vi "Loop.vi"(9 "Error Queue":refnum<queue>, 10 "Event Actor Queue":refnum<queue>, 11 "Dev Actor Panel":refnum<class "Dev Panel.lvclass">) -> ()   [LabVIEW 2021, in "Dev Panel.lvclass"]
uses:
  Dev Panel.lvclass
  C:/git/jettl/src/Event Actor/Event Actor.lvclass
  Actor/Event Actor/Event Actor.lvclass
  Dev Panel.lvclass/Dev Panel.ctl
  Actor/Msgs/Teardown/Teardown Msg/Teardown Msg.lvclass
  C:/git/jettl/src/Actor/Msg/Msg.lvclass
  Msgs/Pop Up/Pop Up Msg/Pop Up Msg.lvclass
  Actor/Msgs/Merge Error/Merge Error Msg/Merge Error Msg.lvclass
panel:
  in  "Button":bool
  out "String Indicator":string
  in  "Pop Up":bool
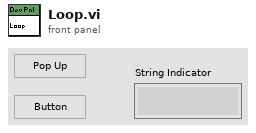
[diagram p1: front panel]
types:
  T1 = cluster{"Teardown":refnum<user-event>, "Pop Up":refnum<user-event>, "String Indicator":refnum<user-event>, "Button":refnum<user-event>}
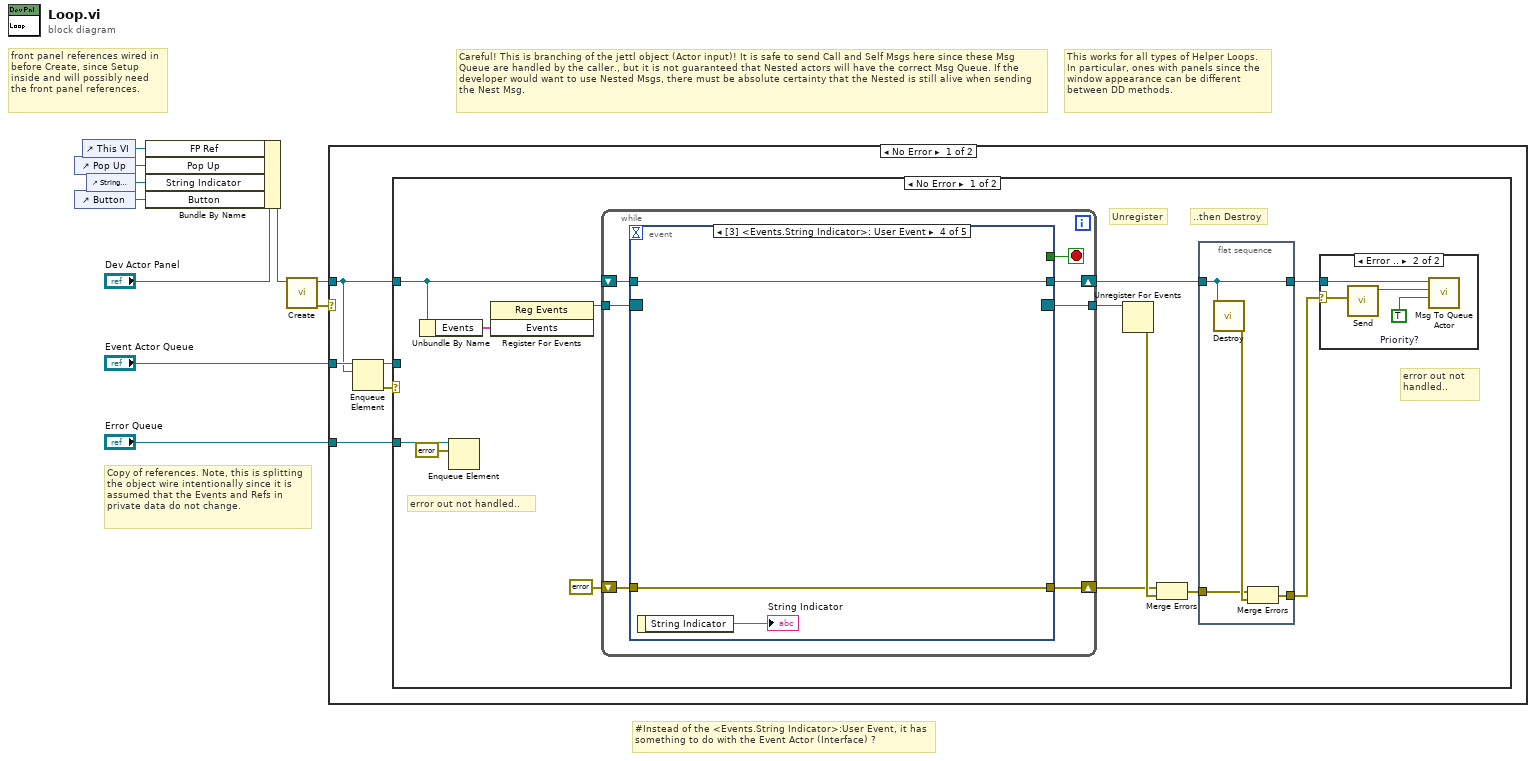
[diagram p0: block diagram]
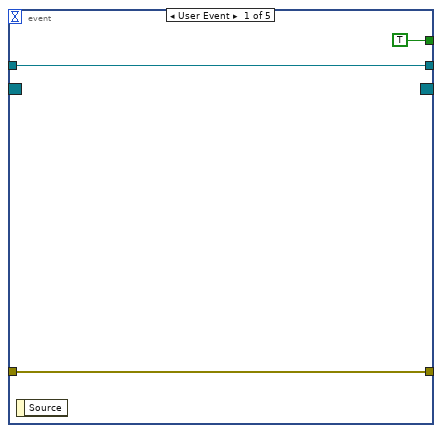
[diagram p3: hidden frame]
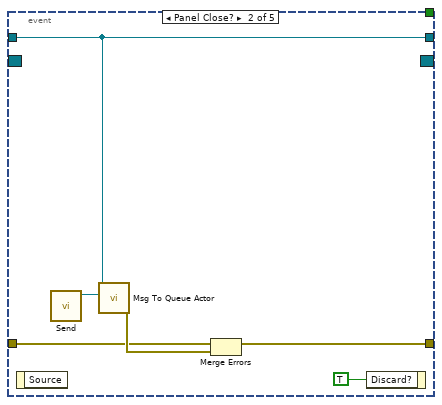
[diagram p4: hidden frame]
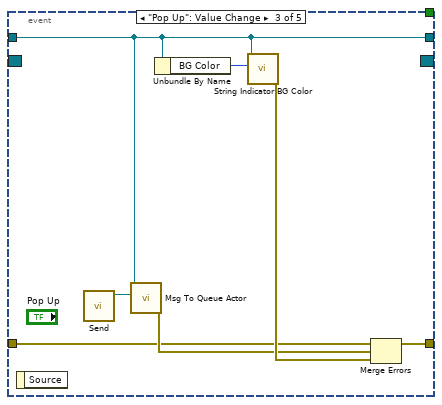
[diagram p5: hidden frame]
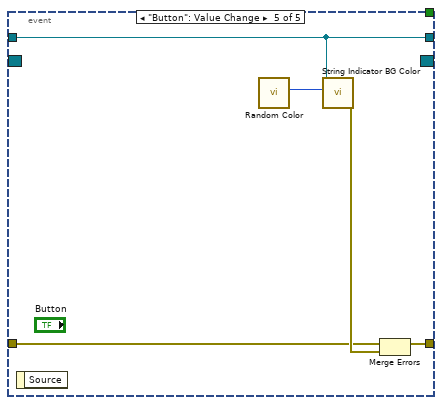
[diagram p6: hidden frame]
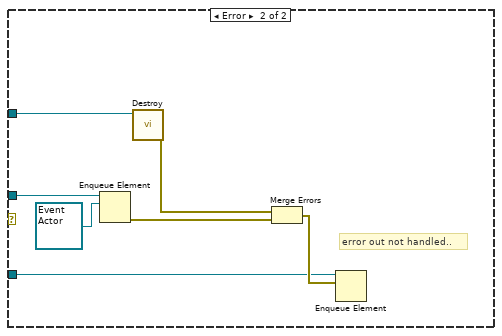
[diagram p7: hidden frame]
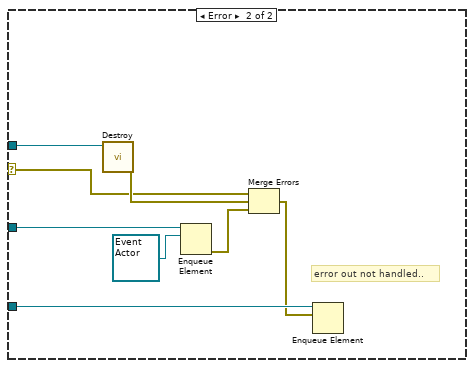
[diagram p8: hidden frame]
diagram:
  # "#Instead of the <Events.String Indicator>:User Event, it has something to do with the Event Actor (Interface) ?"
  # "Copy of references. Note, this is splitting the object wire intentionally since it is assumed that the Events and Refs in private data do not change."
  # "front panel references wired in before Create, since Setup inside and will possibly need the front panel references."
  # "This works for all types of Helper Loops. In particular, ones with panels since the window appearance can be different between DD methods."
  # "Careful! This is branching of the jettl object (Actor input)! It is safe to send Call and Self Msgs here since these Msg Queue are handled by the caller., but it is not guaranteed that Nested actors will have the correct Msg Queue. If the developer would want to use Nested Msgs, there must be absolute certainty that the Nested is still alive when sending the Nest Msg."
  n1 = control-ref of="Pop Up"() -> (w8:refnum<vi>)
  n2 = control-ref of="Button"() -> (w7:refnum<vi>)
  n3 = control-ref of="This VI"() -> (w2:refnum<vi>)
  n4 = control-ref of="String Indicator"() -> (w9:refnum<vi>)
  n5 = Bundle By Name(cluster="Dev Actor Panel", "FP Ref"=w2, "Pop Up"=w8, "String Indicator"=w9, "Button"=w7) -> (w3:refnum<class "Dev Panel.lvclass">)
  n6 = call "Create.vi"("Dev Actor Panel in"=w3) -> ("error out"=w10:errorcluster, "Dev Actor Panel out"=w4:refnum<class "Dev Panel.lvclass">)  [unwired: 9 in]
  n7 = case shown="No Error" w10 {
    selector: w10 -> [_ w80]
    tunnel: w4 -> [w13 w82]
    tunnel: "Error Queue" -> [w15 w79]
    tunnel: "Event Actor Queue" -> [w14 w77]
    frame No Error {
      n8 = Enqueue Element(queue=w14, element=w13) -> (queue out=w11:refnum<queue>, error out=w12:errorcluster)  [unwired: 2 in, 1 out]
      n9 = case shown="No Error" w12 {
        tunnel: w15 -> [w19 w70]
        tunnel: w13 -> [w17 w68]
        tunnel: w11 -> [_ w69]
        frame No Error {
          # "error out not handled.."
          # "error out not handled.."
          # "..then Destroy"
          # "Unregister"
          n10 = Unbundle By Name(w17) -> ("Events"=w26:T1)
          n11 = Enqueue Element(queue=w19, element=errorcluster {"status"=FALSE, "code"=0, "source"=""}) -> ()  [unwired: 2 in, 3 out]
          n12 = register-events ("Main Register for Events")(w26) -> (reference out=w27:refnum<event-registration>)  [unwired: 2 in, 1 out]
          n13 = while {
            shift-right: [w40] -> w22
            shift-left: w17 -> [w39]
            tunnel: w27 -> [w43]
            tunnel: [w41] -> w28
            shift-right: [w38] -> w23
            shift-left: errorcluster {"status"=FALSE, "code"=0, "source"=""} ("error out") -> [w37]
            stop <- w42 stop-if-true
            n14 = event "UI Events" shown="[3] <Events.String Indicator>: User Event" {
              selector: w43 -> [_ _ _ _ _]
              dyn-events: [_ _ _ _ _] -> w41
              timeout: _ -> [_ _ _ _ _]
              tunnel: [TRUE _ _ _ _] -> w42
              tunnel: [w45 w50 w56 w62 w67] -> w40
              tunnel: w39 -> [w45 w50 w56 w62 w67]
              tunnel: [w44 w51 w59 w61 w66] -> w38
              tunnel: w37 -> [w44 w47 w53 w61 w64]
              event User Event {
                n15 = event-data() -> ()  [unwired: 1 in, 1 out]
              }
              event Panel Close? {
                n16 = event-data() -> ()  [unwired: 1 in, 1 out]
                n17 = call "Send.vi"() -> ("Teardown Msg out"=w49:refnum<class "Teardown Msg.lvclass">)  [unwired: 11 in]
                n18 = call-dynamic "Msg To Queue Actor.vi"("Msg"=w49, "Dev Panel in"=w50) -> ("error out"=w48:errorcluster)  [unwired: 9 in]
                n19 = Merge Errors(w47, w48) -> (w51:errorcluster)
                n20 = event-data("Discard?"=TRUE) -> ()  [unwired: 1 in, 1 out]
              }
              event "Pop Up": Value Change {
                n21 = event-data() -> ()  [unwired: 1 in, 1 out]
                n22 = call "Send.vi"() -> ("Pop Up Msg out"=w55:refnum<class "Pop Up Msg.lvclass">)  [unwired: 11 in]
                n23 = call-dynamic "Msg To Queue Actor.vi"("Msg"=w55, "Dev Panel in"=w56) -> ("error out"=w54:errorcluster)  [unwired: 9 in]
                n24 = Unbundle By Name(w56) -> ("BG Color"=w57:u32)
                n25 = call "String Indicator BG Color.vi"("BG Color"=w57, "Dev Panel in"=w56) -> ("error out"=w58:errorcluster)  [unwired: 9 in]
                n26 = Merge Errors(w53, w54, w58) -> (w59:errorcluster)
              }
              event User Event {
                n27 = event-data() -> ("String Indicator"=→"String Indicator":string)  [unwired: 1 in]
              }
              event "Button": Value Change {
                n28 = event-data() -> ()  [unwired: 1 in, 1 out]
                n29 = call "Random Color.vi"() -> ("Color"=w63:u32)  [unwired: 11 in]
                n30 = call "String Indicator BG Color.vi"("BG Color"=w63, "Dev Panel in"=w67) -> ("error out"=w65:errorcluster)  [unwired: 9 in]
                n31 = Merge Errors(w64, w65) -> (w66:errorcluster)
              }
            }
          }
          n32 = Unregister For Events(event registration refnum=w28) -> (error out=w24:errorcluster)  [unwired: 1 in]
          n33 = Merge Errors(w23, w24) -> (w21:errorcluster)
          n34 = flat-sequence {
            tunnel: w22 -> [w33]
            tunnel: [w36] -> w20
            tunnel: w21 -> [w34]
            tunnel: [w33] -> w16
            frame #0 {
              n35 = call "Destroy.vi"("Dev Actor Panel in"=w33) -> ("error out"=w35:errorcluster)  [unwired: 10 in]
              n36 = Merge Errors(w34, w35) -> (w36:errorcluster)
            }
          }
          n37 = case shown="Error .." w20 {
            selector: w20 -> [_ w32]
            tunnel: w16 -> [_ w31]
            frame No Error {
            }
            frame Error {
              w29 = TRUE  # Priority?
              n38 = call "Send.vi"("Error"=w32) -> ("Merge Error Msg out"=w30:refnum<class "Merge Error Msg.lvclass">)  [unwired: 10 in]
              n39 = call-dynamic "Msg To Queue Actor.vi"("Priority?"=w29, "Msg"=w30, "Dev Panel in"=w31) -> ()  [unwired: 8 in, 1 out]
            }
          }
        }
        frame Error {
          # "error out not handled.."
          n40 = Enqueue Element(queue=w69, element=refnum<class "Event Actor.lvclass"> refnum) -> (error out=w71:errorcluster)  [unwired: 2 in, 2 out]
          n41 = call "Destroy.vi"("Dev Actor Panel in"=w68) -> ("error out"=w74:errorcluster)  [unwired: 10 in]
          n42 = Merge Errors(w74, w71) -> (w73:errorcluster)
          n43 = Enqueue Element(queue=w70, element=w73) -> ()  [unwired: 2 in, 3 out]
        }
      }
    }
    frame Error {
      # "error out not handled.."
      n44 = call "Destroy.vi"("Dev Actor Panel in"=w82) -> ("error out"=w81:errorcluster)  [unwired: 10 in]
      n45 = Enqueue Element(queue=w77, element=refnum<class "Event Actor.lvclass"> refnum) -> (error out=w75:errorcluster)  [unwired: 2 in, 2 out]
      n46 = Merge Errors(w80, w81, w75) -> (w78:errorcluster)
      n47 = Enqueue Element(queue=w79, element=w78) -> ()  [unwired: 2 in, 3 out]
    }
  }
